vi "Subvi_Training_Baseline_w_range_w_weight.vi"(4 "Nontarget_Flash_Order":i32[][](array[numeric]), 5 "Target_Flash_Order":i64[](array[numeric]), 6 "samples per channel":i32=25, 7 "Brain_data_source":dbl[](array[numeric]) caption="EEG_Raw_Data" format="%0.3f", 8 "rate":dbl=500.0 caption="Rate" format="%0.2f", 9 "Experimentation_num":i32=2, 10 "Random_num":i32=9, 11 "Random_Repeat":i32=20) -> (0 "Target_ERP":dbl[](array[numeric]), 1 "NonTarget":dbl[][](array[numeric]), 2 "Nontarget_ERP":dbl[](array[numeric]), 3 "Target":dbl[][](array[numeric]))   [LabVIEW 2014]
uses:
  <vilib>/Analysis/3filter.llb/Filter Passband Type.ctl
  <vilib>/Analysis/baseanly.llb/Mean (DBL).vi
  <vilib>/Analysis/3filter.llb/Butterworth Filter (DBL).vi
  <vilib>/Analysis/NI_AALBase.lvlib
  <vilib>/Utility/file.llb/Read From Spreadsheet File (DBL).vi
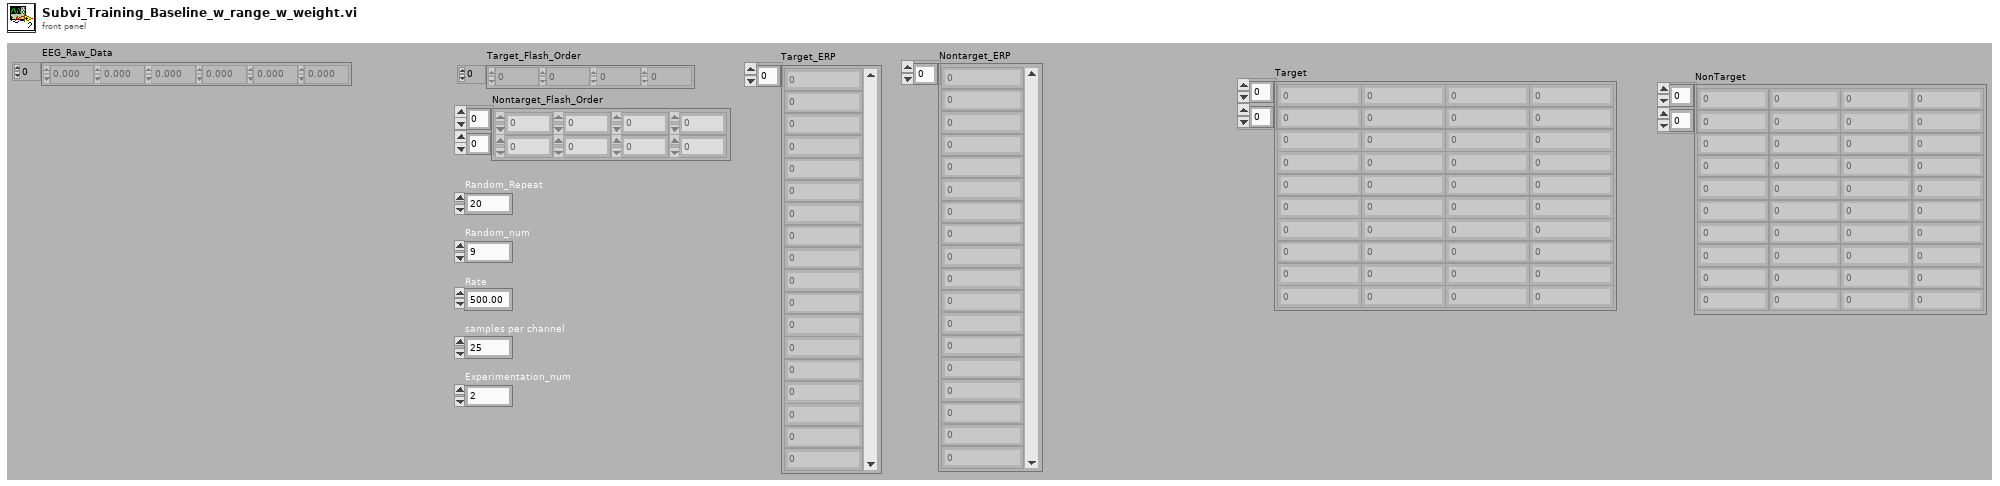
[diagram p1: front panel]
types:
  T1 = typedef "NI_AALBase.lvlib/Filter Passband Type.ctl" = enum32{"Lowpass", "Highpass", "Bandpass", "Bandstop"}
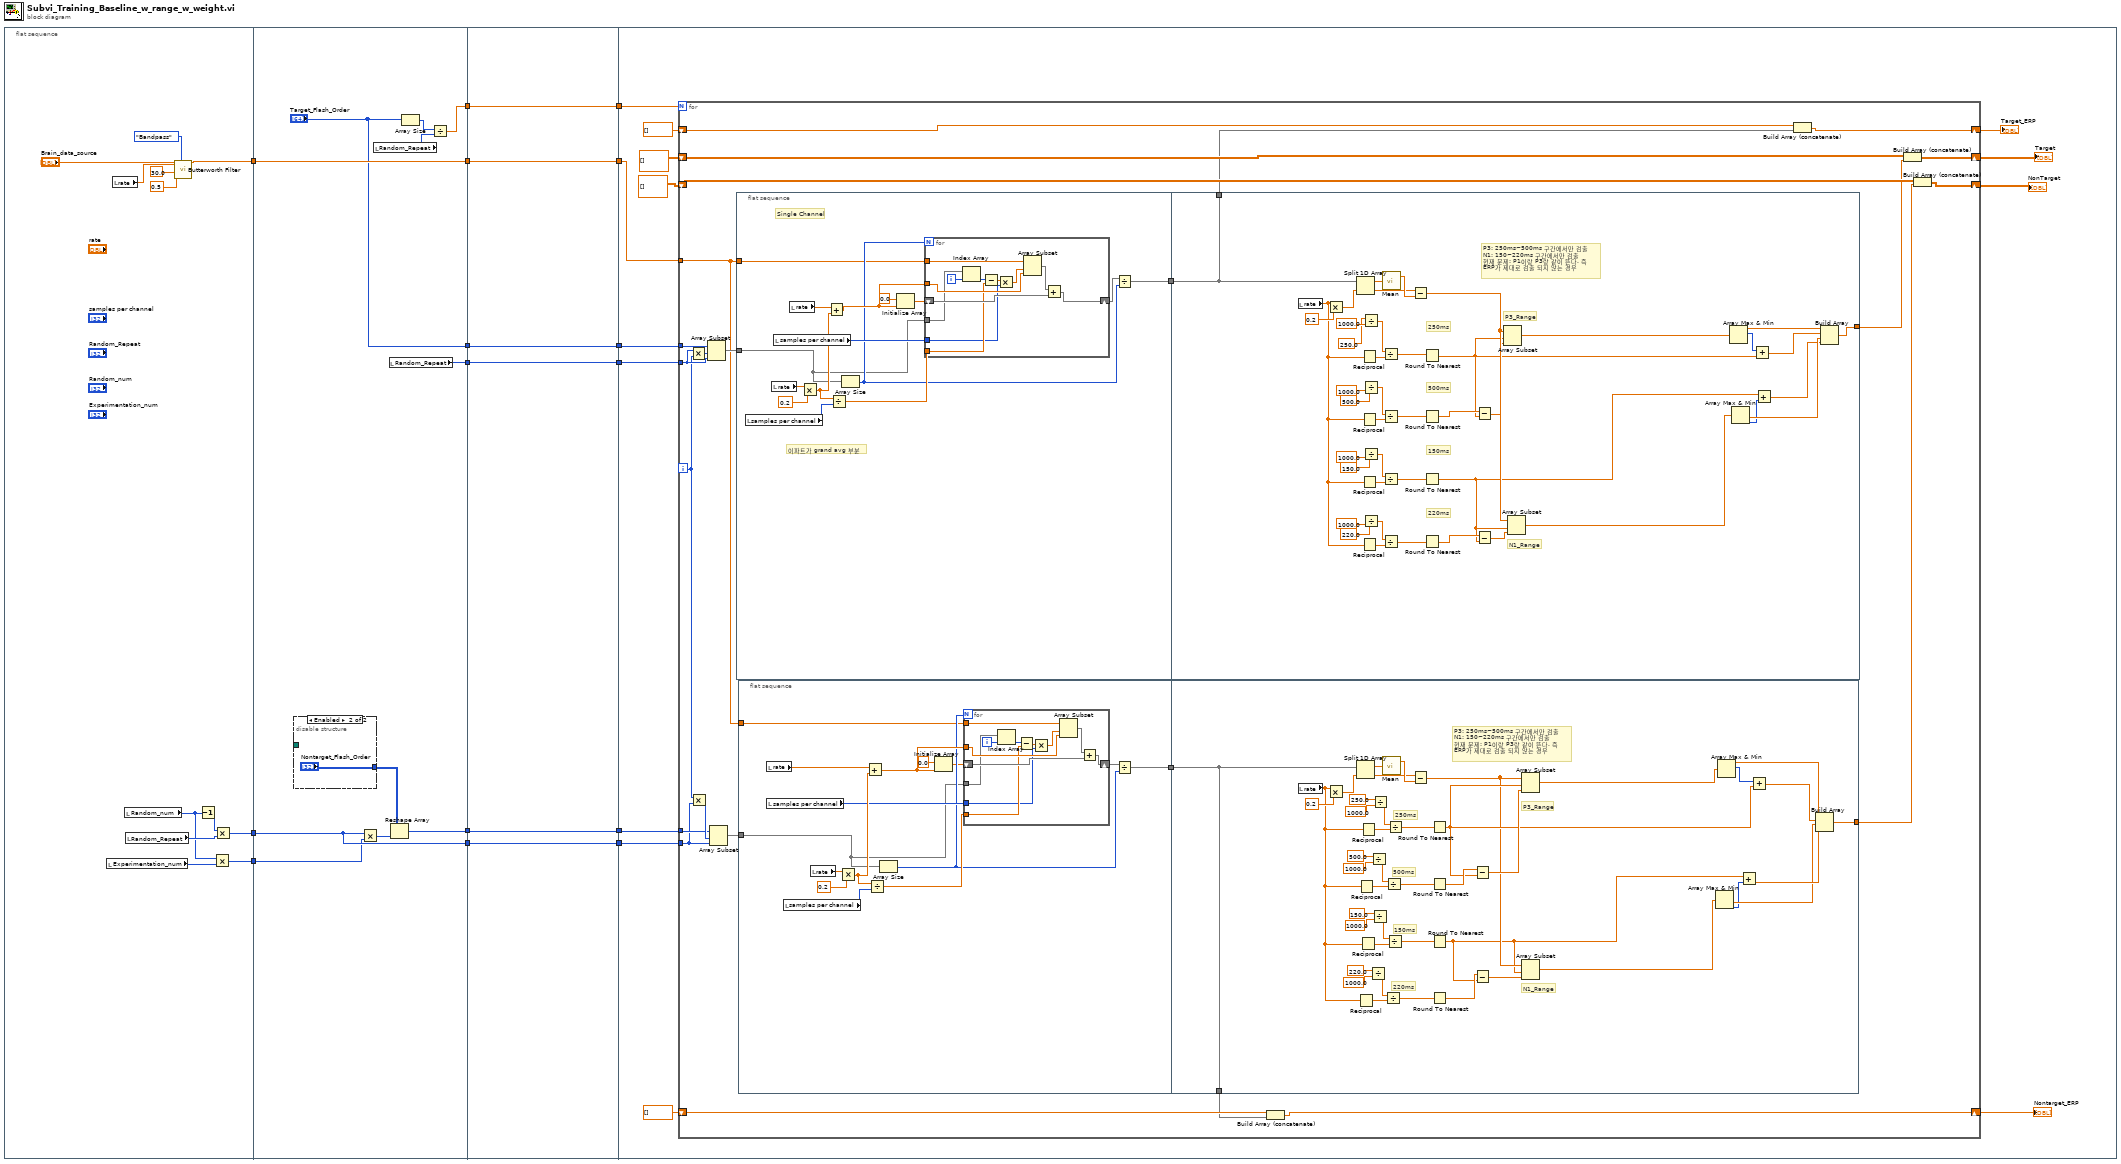
[diagram p0: block diagram]
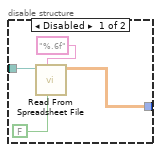
[diagram p2: hidden frame]
diagram:
  n1 = flat-sequence {
    tunnel: [w16] -> w15
    tunnel: [w25] -> w14
    tunnel: [w22] -> w13
    tunnel: w15 -> [w38]
    tunnel: [w38] -> w12
    tunnel: [w35] -> w10
    tunnel: ["Target_Flash_Order"] -> w8
    tunnel: [w34] -> w6
    tunnel: w14 -> [w31]
    tunnel: [w32] -> w4
    tunnel: [w31] -> w2
    tunnel: w13 -> [w30]
    tunnel: w12 -> [w44]
    tunnel: [w44] -> w11
    tunnel: w10 -> [w49]
    tunnel: [w49] -> w9
    tunnel: w8 -> [w48]
    tunnel: [w48] -> w7
    tunnel: w6 -> [w47]
    tunnel: [w47] -> w5
    tunnel: w4 -> [w46]
    tunnel: [w46] -> w3
    tunnel: w2 -> [w45]
    tunnel: [w45] -> w1
    tunnel: w11 -> [w63]
    tunnel: w9 -> [w54]
    tunnel: w7 -> [w62]
    tunnel: w5 -> [w61]
    tunnel: w3 -> [w60]
    tunnel: w1 -> [w59]
    frame #0 {
      n2 = local read "Experimentation_num"() -> (w24:i32)
      n3 = local read "rate"() -> (w18:dbl)
      n4 = local read "Random_num"() -> (w23:i32)
      n5 = local read "Random_Repeat"() -> (w26:i32)
      n6 = call-poly <vilib>:"Butterworth Filter.vi"("filter type"=Filter_Passband_Type."Bandpass", "low cutoff freq: fl"=0.5, "high cutoff freq: fh"=30.0, "sampling freq: fs"=w18, "X"="Brain_data_source") -> ("Filtered X"=w16:dbl[])  [unwired: 3 in, 1 out]
      n7 = Decrement(x=w23) -> (x-1=w27:i32)
      n8 = Multiply(x=w23, y=w24) -> (x*y=w22:i32)
      n9 = Multiply(x=w27, y=w26) -> (x*y=w25:i32)
    }
    frame #1 {
      n10 = disable-structure shown="Enabled" {
        disable-tunnel: _ -> [w42 _]
        disable-tunnel: [w40 "Nontarget_Flash_Order"] -> w29
        frame Disabled {
          n11 = call-poly <vilib>:"Read From Spreadsheet File.vi"("transpose (no:F)"=FALSE, "format (%.3f)"="%.6f", "file path (dialog if empty)"=w42) -> ("all rows"=w40:dbl[][])  [unwired: 4 in, 4 out]
        }
        frame Enabled {
        }
      }
      n12 = Multiply(x=w31, y=w30) -> (x*y=w33:i32)
      n13 = local read "Random_Repeat"() -> (w36:i32)
      n14 = local read "Random_Repeat"() -> (w34:i32)
      n15 = Reshape Array(w29, w33) -> (w32:i32[])
      n16 = Array Size(array="Target_Flash_Order") -> (size(s)=w37:i32)
      n17 = Divide(x=w37, y=w36) -> (x/y=w35:dbl)
    }
    frame #2 {
    }
    frame #3 {
      n18 = for {
        N: w54 -> [_]
        tunnel: w63 -> [w83]
        tunnel: w62 -> [w87]
        tunnel: w61 -> [w85]
        tunnel: w60 -> [w80]
        tunnel: w59 -> [w78]
        shift-right: [w76] -> w56
        shift-left: dbl[][] [] -> [w77]
        shift-right: [w75] -> w55
        shift-left: dbl[][] [] -> [w74]
        shift-right: [w70] -> w51
        shift-left: dbl[] [] -> [w68]
        shift-right: [w71] -> w50
        shift-left: dbl[] [] -> [w73]
        i -> [w81]
        n19 = Multiply(x=w85, y=w81) -> (x*y=w86:i32)
        n20 = Multiply(x=w81, y=w78) -> (x*y=w82:i32)
        n21 = Array Subset(array=w87, index=w86, length=w85) -> (w84:i64[])
        n22 = Array Subset(array=w80, index=w82, length=w78) -> (w79:i32[])
        n23 = flat-sequence {
          tunnel: w83 -> [w159]
          tunnel: w84 -> [w163]
          tunnel: [w158] -> w67
          tunnel: [w223] -> w65
          tunnel: [w185] -> w69
          tunnel: w67 -> [w185]
          frame #0 {
            # "Single Channel"
            # "이파트가 grand avg 부분"
            n24 = local read "samples per channel"() -> (w166:i32)
            n25 = local read "rate"() -> (w168:dbl)
            n26 = local read "samples per channel"() -> (w165:i32)
            n27 = local read "rate"() -> (w170:dbl)
            n28 = Multiply(x=w168, y=0.2) -> (x*y=w172:dbl)
            n29 = Add(x=w170, y=w172) -> (x+y=w171:dbl)
            n30 = Divide(x=w172, y=w166) -> (x/y=w169:dbl)
            n31 = Array Size(array=w163) -> (size(s)=w164:i32)
            n32 = Initialize Array(0.0 ("element"), w171) -> (w162:dbl[])
            n33 = for {
              N: w164 -> [_]
              shift-right: [w182] -> w160
              shift-left: w162 -> [w183]
              tunnel: w171 -> [w181]
              tunnel: w163 -> [w179]
              tunnel: w169 -> [w177]
              tunnel: w165 -> [w175]
              tunnel: w159 -> [w174]
              i -> [w180]
              n34 = Index Array(array=w179, index=w180) -> (element=w178:i64)
              n35 = Subtract(x=w178, y=w177) -> (x-y=w176:dbl)
              n36 = Multiply(x=w176, y=w175) -> (x*y=w184:dbl)
              n37 = Array Subset(array=w174, index=w184, length=w181) -> (w173:dbl[])
              n38 = Add(x=w173, y=w183) -> (x+y=w182:dbl[])
            }
            n39 = Divide(x=w160, y=w164) -> (x/y=w158:dbl[])
          }
          frame #1 {
            # "N1_Range"
            # "P3_Range"
            # "220ms"
            # "150ms"
            # "500ms"
            # "250ms"
            # "P3: 250ms~500ms 구간에서만 검출\nN1: 150~220ms 구간에서만 검출\n현재 문제: P1이랑 P3랑 같이 뜬다. 즉\nERP가 제대로 검출 되지 않는 경우"
            n40 = local read "rate"() -> (w215:dbl)
            n41 = Multiply(x=w215, y=0.2) -> (x*y=w221:dbl)
            n42 = Split 1D Array(array=w185, index=w221) -> (first subarray=w220:dbl[], second subarray=w216:dbl[])
            n43 = Reciprocal(x=w215) -> (1/x=w214:dbl)
            n44 = Reciprocal(x=w215) -> (1/x=w213:dbl)
            n45 = Reciprocal(x=w215) -> (1/x=w212:dbl)
            n46 = Reciprocal(x=w215) -> (1/x=w211:dbl)
            n47 = Divide(x=250.0, y=1000.0) -> (x/y=w210:dbl)
            n48 = Divide(x=500.0, y=1000.0) -> (x/y=w209:dbl)
            n49 = Divide(x=150.0, y=1000.0) -> (x/y=w208:dbl)
            n50 = Divide(x=220.0, y=1000.0) -> (x/y=w207:dbl)
            n51 = call-poly <vilib>:"Mean.vi"("X"=w220) -> ("mean"=w219:dbl)  [unwired: 1 out]
            n52 = Divide(x=w210, y=w214) -> (x/y=w198:dbl)
            n53 = Divide(x=w209, y=w213) -> (x/y=w197:dbl)
            n54 = Divide(x=w208, y=w212) -> (x/y=w196:dbl)
            n55 = Divide(x=w207, y=w211) -> (x/y=w195:dbl)
            n56 = Subtract(x=w216, y=w219) -> (x-y=w192:dbl[])
            n57 = Round To Nearest(number=w198) -> (nearest integer value=w191:dbl)
            n58 = Round To Nearest(number=w197) -> (nearest integer value=w194:dbl)
            n59 = Round To Nearest(number=w196) -> (nearest integer value=w189:dbl)
            n60 = Round To Nearest(number=w195) -> (nearest integer value=w193:dbl)
            n61 = Subtract(x=w194, y=w191) -> (x-y=w190:dbl)
            n62 = Subtract(x=w193, y=w189) -> (x-y=w188:dbl)
            n63 = Array Subset(array=w192, index=w191, length=w190) -> (w187:dbl[])
            n64 = Array Subset(array=w192, index=w189, length=w188) -> (w186:dbl[])
            n65 = Array Max & Min(array=w187) -> (max value=w227:dbl, max index (indices)=w218:i32)  [unwired: 2 out]
            n66 = Array Max & Min(array=w186) -> (min value=w225:dbl, min index (indices)=w217:i32)  [unwired: 2 out]
            n67 = Add(x=w218, y=w191) -> (x+y=w226:dbl)
            n68 = Add(x=w189, y=w217) -> (x+y=w224:dbl)
            n69 = Build Array(w227, w226, w225, w224) -> (w223:dbl[])
          }
        }
        n70 = flat-sequence {
          tunnel: w83 -> [w89]
          tunnel: w79 -> [w93]
          tunnel: [w88] -> w66
          tunnel: [w153] -> w64
          tunnel: [w115] -> w72
          tunnel: w66 -> [w115]
          frame #0 {
            n71 = local read "rate"() -> (w100:dbl)
            n72 = local read "samples per channel"() -> (w95:i32)
            n73 = local read "samples per channel"() -> (w96:i32)
            n74 = local read "rate"() -> (w98:dbl)
            n75 = Multiply(x=w98, y=0.2) -> (x*y=w102:dbl)
            n76 = Add(x=w100, y=w102) -> (x+y=w101:dbl)
            n77 = Divide(x=w102, y=w96) -> (x/y=w99:dbl)
            n78 = Array Size(array=w93) -> (size(s)=w94:i32)
            n79 = Initialize Array(0.0 ("element"), w101) -> (w92:dbl[])
            n80 = for {
              N: w94 -> [_]
              shift-right: [w112] -> w90
              shift-left: w92 -> [w113]
              tunnel: w101 -> [w111]
              tunnel: w93 -> [w109]
              tunnel: w99 -> [w107]
              tunnel: w95 -> [w105]
              tunnel: w89 -> [w104]
              i -> [w110]
              n81 = Index Array(array=w109, index=w110) -> (element=w108:i32)
              n82 = Subtract(x=w108, y=w107) -> (x-y=w106:dbl)
              n83 = Multiply(x=w106, y=w105) -> (x*y=w114:dbl)
              n84 = Array Subset(array=w104, index=w114, length=w111) -> (w103:dbl[])
              n85 = Add(x=w103, y=w113) -> (x+y=w112:dbl[])
            }
            n86 = Divide(x=w90, y=w94) -> (x/y=w88:dbl[])
          }
          frame #1 {
            # "N1_Range"
            # "P3_Range"
            # "220ms"
            # "150ms"
            # "500ms"
            # "250ms"
            # "P3: 250ms~500ms 구간에서만 검출\nN1: 150~220ms 구간에서만 검출\n현재 문제: P1이랑 P3랑 같이 뜬다. 즉\nERP가 제대로 검출 되지 않는 경우"
            n87 = local read "rate"() -> (w129:dbl)
            n88 = Multiply(x=w129, y=0.2) -> (x*y=w151:dbl)
            n89 = Split 1D Array(array=w115, index=w151) -> (first subarray=w150:dbl[], second subarray=w148:dbl[])
            n90 = Reciprocal(x=w129) -> (1/x=w133:dbl)
            n91 = Reciprocal(x=w129) -> (1/x=w141:dbl)
            n92 = Reciprocal(x=w129) -> (1/x=w137:dbl)
            n93 = Reciprocal(x=w129) -> (1/x=w145:dbl)
            n94 = Divide(x=220.0, y=1000.0) -> (x/y=w130:dbl)
            n95 = Divide(x=500.0, y=1000.0) -> (x/y=w138:dbl)
            n96 = Divide(x=150.0, y=1000.0) -> (x/y=w134:dbl)
            n97 = Divide(x=250.0, y=1000.0) -> (x/y=w142:dbl)
            n98 = call-poly <vilib>:"Mean.vi"("X"=w150) -> ("mean"=w149:dbl)  [unwired: 1 out]
            n99 = Divide(x=w130, y=w133) -> (x/y=w125:dbl)
            n100 = Divide(x=w138, y=w141) -> (x/y=w127:dbl)
            n101 = Divide(x=w134, y=w137) -> (x/y=w126:dbl)
            n102 = Divide(x=w142, y=w145) -> (x/y=w128:dbl)
            n103 = Subtract(x=w148, y=w149) -> (x-y=w118:dbl[])
            n104 = Round To Nearest(number=w128) -> (nearest integer value=w122:dbl)
            n105 = Round To Nearest(number=w127) -> (nearest integer value=w124:dbl)
            n106 = Round To Nearest(number=w126) -> (nearest integer value=w116:dbl)
            n107 = Round To Nearest(number=w125) -> (nearest integer value=w119:dbl)
            n108 = Subtract(x=w124, y=w122) -> (x-y=w123:dbl)
            n109 = Subtract(x=w119, y=w116) -> (x-y=w120:dbl)
            n110 = Array Subset(array=w118, index=w122, length=w123) -> (w121:dbl[])
            n111 = Array Subset(array=w118, index=w116, length=w120) -> (w117:dbl[])
            n112 = Array Max & Min(array=w117) -> (min value=w154:dbl, min index (indices)=w147:i32)  [unwired: 2 out]
            n113 = Array Max & Min(array=w121) -> (max value=w157:dbl, max index (indices)=w146:i32)  [unwired: 2 out]
            n114 = Add(x=w116, y=w147) -> (x+y=w155:dbl)
            n115 = Add(x=w146, y=w122) -> (x+y=w156:dbl)
            n116 = Build Array(w157, w156, w154, w155) -> (w153:dbl[])
          }
        }
        n117 = Build Array (concatenate)(w73, w72) -> (w71:dbl[])
        n118 = Build Array (concatenate)(w68, w69) -> (w70:dbl[])
        n119 = Build Array (concatenate)(w77, w65) -> (w76:dbl[][])
        n120 = Build Array (concatenate)(w74, w64) -> (w75:dbl[][])
      }
      "Target" <- w56
      "NonTarget" <- w55
      "Target_ERP" <- w51
      "Nontarget_ERP" <- w50
    }
  }
